vi "init_runner_maze_start.vi"(7 "maze array":bool[][](array[boolean])) -> (8 "maze with runner array":T1[][](array[typedef]))   [LabVIEW 2016]
doc: "Initializes the maze array with an open cell of the mouse and returns the maze with runner array.\n\nMuhannad Alghamdi\nCSUSB Physics 350"
uses:
  typedefs/cell_typedef.ctl
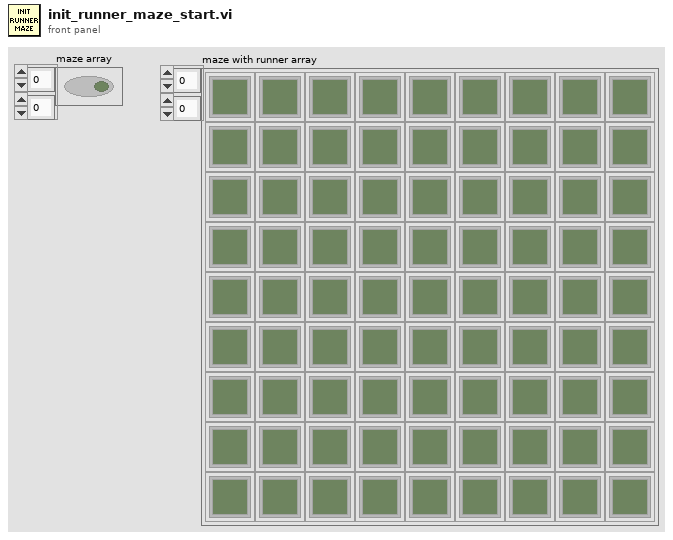
[diagram p1: front panel]
types:
  T1 = typedef "cell_typedef.ctl" = cluster{"open":bool, "runner":u16}
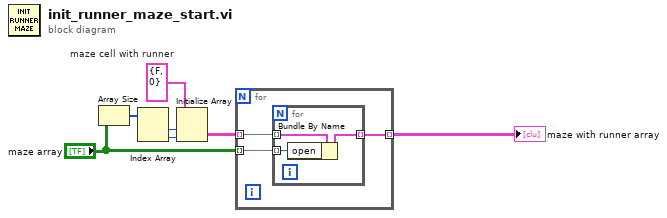
[diagram p0: block diagram]
diagram:
  w5 = T1 {"open"=FALSE, "runner"=0}  # maze cell with runner
  n1 = Array Size(array="maze array") -> (size(s)=w2:i32[])
  n2 = Index Array(array=w2) -> (element #1=w3:i32, element #2=w4:i32)  [unwired: 2 in]
  n3 = Initialize Array(w5, w3, w4) -> (w7:T1[][])
  n4 = for {
    tunnel: w7 -> [w10] mode=indexing
    tunnel: "maze array" -> [w9] mode=indexing
    tunnel: [w8] -> w1 mode=indexing
    n5 = for {
      tunnel: w10 -> [w13] mode=indexing
      tunnel: w9 -> [w12] mode=indexing
      tunnel: [w11] -> w8 mode=indexing
      n6 = Bundle By Name(cluster=w13, "open"=w12) -> (w11:T1)
    }
  }
  "maze with runner array" <- w1
